vi "写入命令类.lvclass.vi"(8 "error in (no error)":errorcluster caption="错误输入（无错误）", 10 "命令类.lvclass":refnum<class "命令类.lvclass">, 11 "控制盒输入":refnum<class "控制盒.lvclass">) -> (0 "error out":errorcluster caption="错误输出", 3 "控制盒输出":refnum<class "控制盒.lvclass">)   [LabVIEW 2011, in "控制盒.lvclass"]
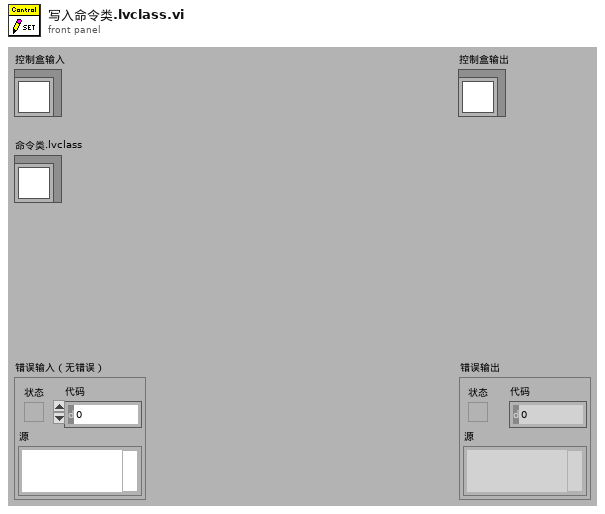
[diagram p1: front panel]
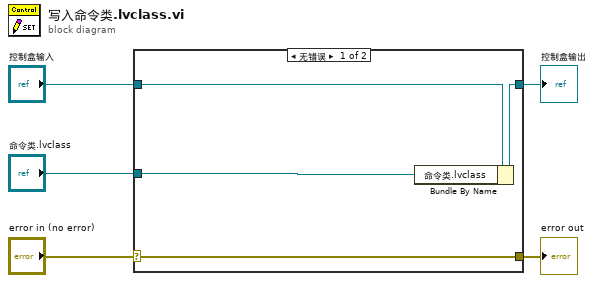
[diagram p0: block diagram]
diagram:
  n1 = case shown="无错误" "error in (no error)" {
    selector: "error in (no error)" -> [w9 w10]
    tunnel: [w9 w10] -> w4
    tunnel: [w7 w11] -> w2
    tunnel: "控制盒输入" -> [w8 w11]
    tunnel: "命令类.lvclass" -> [w6 _]
    frame No Error {
      n2 = Bundle By Name(cluster=w8, "命令类.lvclass"=w6) -> (w7:refnum<class "控制盒.lvclass">)
    }
    frame Error {
    }
  }
  "error out" <- w4
  "控制盒输出" <- w2
